vi "Print Function Description.vi"(8 "error in (no error)":errorcluster, 10 "functionDescription":string, 11 "functionName":string) -> (0 "error out":errorcluster, 2 "functionDescription out":string, 3 "functionName out":string)   [LabVIEW 2009, in "LabVIEWWrapper_PassingDataSampleDLL.lvlib"]
doc: "void PrintFunctionDescription(char *functionName, char *functionDescription);"
uses:
  LabVIEWWrapper_PassingDataSampleDLL.lvlib
  PassingDataSampleDLL.dll
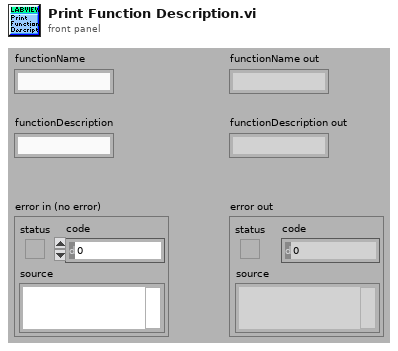
[diagram p1: front panel]
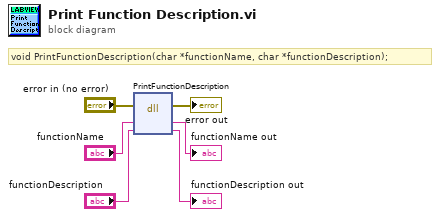
[diagram p0: block diagram]
diagram:
  # "void PrintFunctionDescription(char *functionName, char *functionDescription);"
  n1 = dll-call lib="C:/My Dropbox/Systems Engineering Application/SDK/C Integration/LabVIEWWrapper/PassingDataSampleDLL.*" fn="PrintFunctionDescription"(error in="error in (no error)", "functionName"="functionName", "functionDescription"="functionDescription") -> (error out=→"error out":errorcluster, "functionName"=→"functionName out":string, "functionDescription"=→"functionDescription out":string)  [unwired: 3 in, 1 out]
